vi "Laurel Meter IP Tester.vi"() -> ()   [LabVIEW 2016]
uses:
  Type Definitions/Laurel Serial Commands.ctl
  Type Definitions/Laurel Connection Type.ctl
panel:
  out "Single Item":dbl
  in  "Connection Type":T1
  in  "All Items Byte Count (Flow Rate)":i32=17
  in  "Laurel Serial Commands":T2
  out "return count":i32
  in  "Individual Byte Count":i32=9
  out "Output 6":string="0000.00 0004.71"
  out "Output 5":string="0000.00 0004.71"
  out "Output 4":string="0000.00 0004.71"
  out "Output 3":string="0000.00 0004.71"
  out "Output 2":string="0000.00 0004.71"
  out "Output 1":string="0000.00 0004.71"
  in  "STOP 6":bool
  out "Loop Speed 6":u32
  out "Flow Rate 6":dbl
  in  "Send Command in 8":T3(ring)=enum."Reading: All Active Items"
  out "Gallons 6":dbl
  in  "Error In 7":errorcluster
  out "Error Out 7":errorcluster
  in  "Hot Laurel Only 6":string="10.0.3.169"
  in  "STOP 5":bool
  out "Loop Speed 5":u32
  out "Flow Rate 5":dbl
  out "Gallons 5":dbl
  in  "Error In 6":errorcluster
  out "Error Out 6":errorcluster
  in  "Hot Laurel Only 5":string="10.0.3.167"
  in  "STOP 4":bool
  out "Loop Speed 4":u32
  out "Flow Rate 4":dbl
  in  "Send Command in 6":T3(ring)=enum."Reading: All Active Items"
  out "Gallons 4":dbl
  in  "Error In 5":errorcluster
  out "Error Out 5":errorcluster
  in  "Hot Laurel Only 4":string="10.0.3.165"
  in  "STOP 3":bool
  out "Loop Speed 3":u32
  out "Flow Rate 3":dbl
  in  "Send Command in 5":T3(ring)=enum."Reading: All Active Items"
  out "Gallons 3":dbl
  in  "Error In 4":errorcluster
  out "Error Out 4":errorcluster
  in  "Hot Laurel Only 3":string="10.0.3.163"
  in  "STOP 2":bool
  out "Loop Speed 2":u32
  out "Flow Rate 2":dbl
  in  "Send Command in 4":T3(ring)=enum."Reading: All Active Items"
  out "Gallons 2":dbl
  in  "Error In 3":errorcluster
  out "Error Out 3":errorcluster
  in  "Hot Laurel Only 2":string="10.0.3.161"
  out "Gallons":dbl
  in  "STOP":bool
  out "Loop Speed 1":u32
  out "Flow Rate":dbl
  in  "Send Command in 3":T3(ring)=enum."Reading: All Active Items"
  in  "Error In 2":errorcluster
  out "Error Out 2":errorcluster
  in  "Hot Laurel Only":string="10.0.3.159"
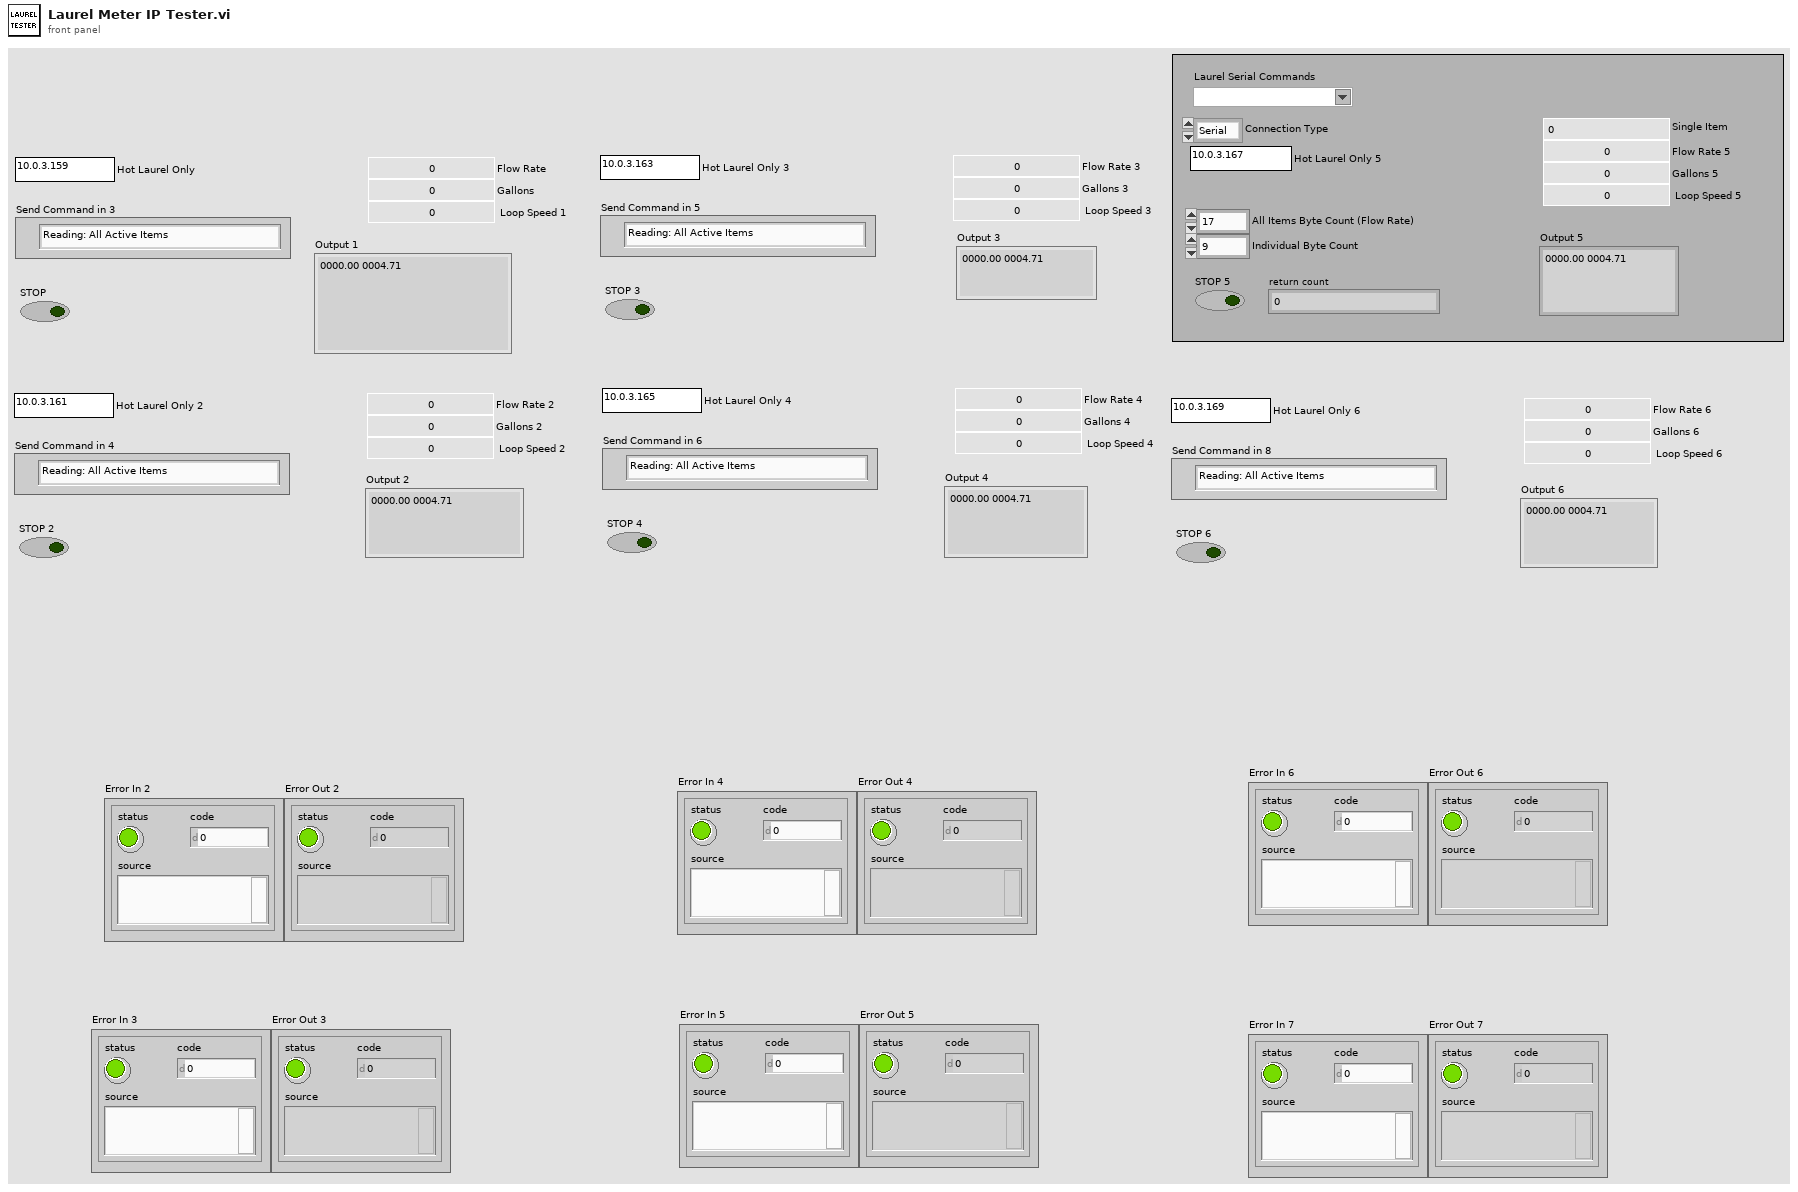
[diagram p1: front panel]
types:
  T1 = typedef "Laurel Connection Type.ctl" = enum16{"Serial", "TCP"}
  T2 = typedef "Laurel Serial Commands.ctl" = string
  T3 = enum16{"Command Mode", "Cold Reset", "Function Reset", "Reading: All Active Items", "Reading: Item 1", "Reading: Item 2", "Reading: Item 3"}
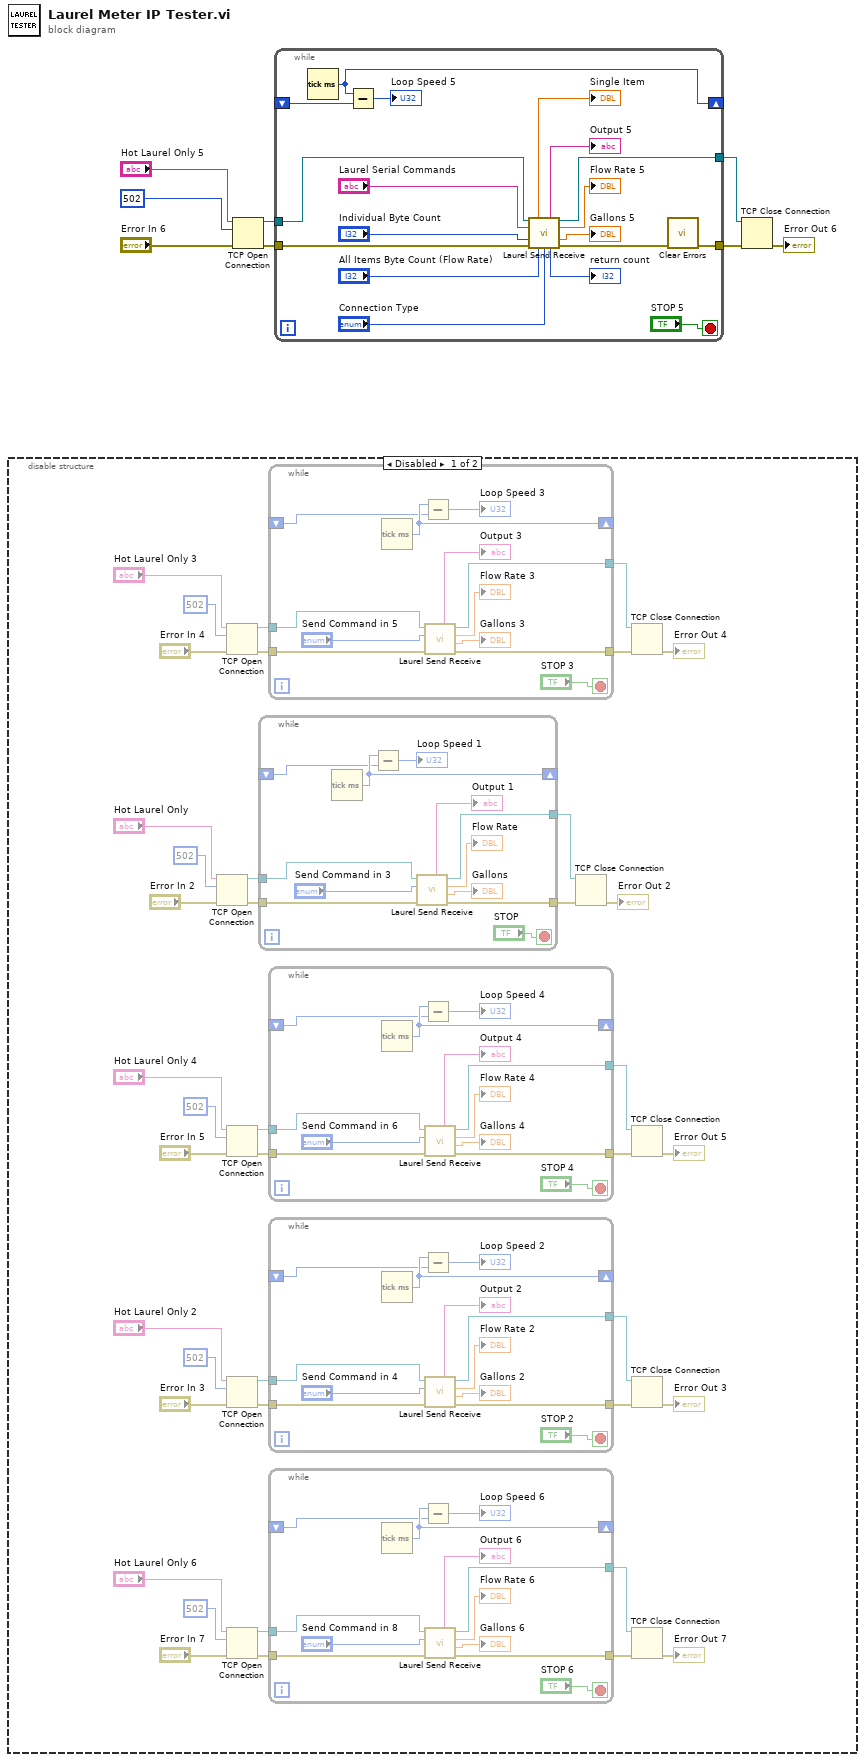
[diagram p0: block diagram]
diagram:
  n1 = disable-structure shown="Disabled" {
    frame Disabled {
      n2 = TCP Open Connection(address="Hot Laurel Only", remote port or service name=u16 502, error in (no error)="Error In 2") -> (connection ID=w45:refnum<k5>, error out=w43:errorcluster)  [unwired: 2 in]
      n3 = TCP Open Connection(address="Hot Laurel Only 3", remote port or service name=u16 502, error in (no error)="Error In 4") -> (connection ID=w29:refnum<k5>, error out=w27:errorcluster)  [unwired: 2 in]
      n4 = TCP Open Connection(address="Hot Laurel Only 4", remote port or service name=u16 502, error in (no error)="Error In 5") -> (connection ID=w20:refnum<k5>, error out=w22:errorcluster)  [unwired: 2 in]
      n5 = TCP Open Connection(address="Hot Laurel Only 2", remote port or service name=u16 502, error in (no error)="Error In 3") -> (connection ID=w36:refnum<k5>, error out=w38:errorcluster)  [unwired: 2 in]
      n6 = TCP Open Connection(address="Hot Laurel Only 6", remote port or service name=u16 502, error in (no error)="Error In 7") -> (connection ID=w12:refnum<k5>, error out=w14:errorcluster)  [unwired: 2 in]
      n7 = while {
        shift-right: [w106] -> _
        shift-left: _ -> [w105]
        tunnel: w43 -> [w102]
        tunnel: [w101] -> w44
        tunnel: w45 -> [w104]
        tunnel: [w103] -> w46
        stop <- "STOP" stop-if-true
        n8 = Tick Count (ms)() -> (millisecond timer value=w106:u32)
        n9 = Subtract(x=w106, y=w105) -> (x-y=→"Loop Speed 1":u32)
        n10 = call "Laurel Send Receive.vi"("error in (no error)"=w102, "Send Command in"="Send Command in 3", "TCP Network Connection in"=w104) -> ("error out"=w101:errorcluster, "Gallons (Item 2)"=→"Gallons":dbl, "Flow Rate (Item 1)"=→"Flow Rate":dbl, "TCP Network Connection out"=w103:refnum<k5>, "Output String"=→"Output 1":string)  [unwired: 2 in, 2 out]
      }
      n11 = while {
        shift-right: [w82] -> _
        shift-left: _ -> [w81]
        tunnel: w27 -> [w78]
        tunnel: [w77] -> w28
        tunnel: w29 -> [w80]
        tunnel: [w79] -> w30
        stop <- "STOP 3" stop-if-true
        n12 = Tick Count (ms)() -> (millisecond timer value=w82:u32)
        n13 = Subtract(x=w82, y=w81) -> (x-y=→"Loop Speed 3":u32)
        n14 = call "Laurel Send Receive.vi"("error in (no error)"=w78, "Send Command in"="Send Command in 5", "TCP Network Connection in"=w80) -> ("error out"=w77:errorcluster, "Gallons (Item 2)"=→"Gallons 3":dbl, "Flow Rate (Item 1)"=→"Flow Rate 3":dbl, "TCP Network Connection out"=w79:refnum<k5>, "Output String"=→"Output 3":string)  [unwired: 2 in, 2 out]
      }
      n15 = while {
        shift-right: [w70] -> _
        shift-left: _ -> [w69]
        tunnel: w22 -> [w66]
        tunnel: [w65] -> w21
        tunnel: w20 -> [w68]
        tunnel: [w67] -> w19
        stop <- "STOP 4" stop-if-true
        n16 = Tick Count (ms)() -> (millisecond timer value=w70:u32)
        n17 = Subtract(x=w70, y=w69) -> (x-y=→"Loop Speed 4":u32)
        n18 = call "Laurel Send Receive.vi"("error in (no error)"=w66, "Send Command in"="Send Command in 6", "TCP Network Connection in"=w68) -> ("error out"=w65:errorcluster, "Gallons (Item 2)"=→"Gallons 4":dbl, "Flow Rate (Item 1)"=→"Flow Rate 4":dbl, "TCP Network Connection out"=w67:refnum<k5>, "Output String"=→"Output 4":string)  [unwired: 2 in, 2 out]
      }
      n19 = while {
        shift-right: [w94] -> _
        shift-left: _ -> [w93]
        tunnel: w38 -> [w90]
        tunnel: [w89] -> w37
        tunnel: w36 -> [w92]
        tunnel: [w91] -> w35
        stop <- "STOP 2" stop-if-true
        n20 = Tick Count (ms)() -> (millisecond timer value=w94:u32)
        n21 = Subtract(x=w94, y=w93) -> (x-y=→"Loop Speed 2":u32)
        n22 = call "Laurel Send Receive.vi"("error in (no error)"=w90, "Send Command in"="Send Command in 4", "TCP Network Connection in"=w92) -> ("error out"=w89:errorcluster, "Gallons (Item 2)"=→"Gallons 2":dbl, "Flow Rate (Item 1)"=→"Flow Rate 2":dbl, "TCP Network Connection out"=w91:refnum<k5>, "Output String"=→"Output 2":string)  [unwired: 2 in, 2 out]
      }
      n23 = while {
        shift-right: [w58] -> _
        shift-left: _ -> [w57]
        tunnel: w14 -> [w54]
        tunnel: [w53] -> w13
        tunnel: w12 -> [w56]
        tunnel: [w55] -> w11
        stop <- "STOP 6" stop-if-true
        n24 = Tick Count (ms)() -> (millisecond timer value=w58:u32)
        n25 = Subtract(x=w58, y=w57) -> (x-y=→"Loop Speed 6":u32)
        n26 = call "Laurel Send Receive.vi"("error in (no error)"=w54, "Send Command in"="Send Command in 8", "TCP Network Connection in"=w56) -> ("error out"=w53:errorcluster, "Gallons (Item 2)"=→"Gallons 6":dbl, "Flow Rate (Item 1)"=→"Flow Rate 6":dbl, "TCP Network Connection out"=w55:refnum<k5>, "Output String"=→"Output 6":string)  [unwired: 2 in, 2 out]
      }
      n27 = TCP Close Connection(connection ID=w46, error in (no error)=w44) -> (error out=→"Error Out 2":errorcluster)  [unwired: 1 in, 1 out]
      n28 = TCP Close Connection(connection ID=w30, error in (no error)=w28) -> (error out=→"Error Out 4":errorcluster)  [unwired: 1 in, 1 out]
      n29 = TCP Close Connection(connection ID=w19, error in (no error)=w21) -> (error out=→"Error Out 5":errorcluster)  [unwired: 1 in, 1 out]
      n30 = TCP Close Connection(connection ID=w35, error in (no error)=w37) -> (error out=→"Error Out 3":errorcluster)  [unwired: 1 in, 1 out]
      n31 = TCP Close Connection(connection ID=w11, error in (no error)=w13) -> (error out=→"Error Out 7":errorcluster)  [unwired: 1 in, 1 out]
    }
    frame Enabled {
    }
  }
  n32 = TCP Open Connection(address="Hot Laurel Only 5", remote port or service name=u16 502, error in (no error)="Error In 6") -> (connection ID=w5:refnum<k5>, error out=w3:errorcluster)  [unwired: 2 in]
  n33 = while {
    shift-right: [w124] -> _
    shift-left: _ -> [w123]
    tunnel: w3 -> [w120]
    tunnel: [w109] -> w4
    tunnel: w5 -> [w122]
    tunnel: [w121] -> w6
    stop <- "STOP 5" stop-if-true
    n34 = Tick Count (ms)() -> (millisecond timer value=w124:u32)
    n35 = Subtract(x=w124, y=w123) -> (x-y=→"Loop Speed 5":u32)
    n36 = call "Laurel Send Receive.vi"("TCP Network Connection in"=w122, "Laurel Serial Commands"="Laurel Serial Commands", "Individual Byte Count"="Individual Byte Count", "error in (no error)"=w120, "All Items Byte Count (Flow Rate)"="All Items Byte Count (Flow Rate)", "Connection Type"="Connection Type") -> ("Single Item"=→"Single Item":dbl, "Output String"=→"Output 5":string, "TCP Network Connection out"=w121:refnum<k5>, "Flow Rate (Item 1)"=→"Flow Rate 5":dbl, "Gallons (Item 2)"=→"Gallons 5":dbl, "return count"=→"return count":i32, "error out"=w110:errorcluster)  [unwired: 2 in, 1 out]
    n37 = call <vilib>:"Clear Errors.vi"("error in (no error)"=w110) -> ("error out"=w109:errorcluster)  [unwired: 5 in, 1 out]
  }
  n38 = TCP Close Connection(connection ID=w6, error in (no error)=w4) -> (error out=→"Error Out 6":errorcluster)  [unwired: 1 in, 1 out]
